vi "Tool Object.vi"(8 "error in (no error)":errorcluster, 11 "Tool Dots in":refnum<class "Tool Dots.lvclass">) -> (0 "error out":errorcluster, 3 "Tool Dots out":refnum<class "Tool Dots.lvclass">)   [LabVIEW 2019, in "Tool Dots.lvclass"]
uses:
  Tool Dots.lvclass
  Settings/ObjectSettings/ObjectSettings.lvclass/ObjectSettings.ctl
  Parse/PathCommands/Point.ctl
  Parse/Dot/Dot.lvclass/Dot.ctl
  Settings/Dot Settings/Dot Settings.lvclass/Dot Settings.ctl
  Parse/Dot/Read cx.vi
  Parse/Dot/Read cy.vi
  Settings/Dot Settings/Dot Settings.lvclass
  C:/Users/Albro/Documents/GitHub/AFM-Lithography/lvsrc/Classes/Settings/ObjectSettings/ObjectSettings.lvclass
  Tool Object/Tool Object.lvclass
  Parse/Dot/Dot.lvclass
  Parse/PathCommands/PathCommands.lvclass
  Settings/ObjectSettings/ObjectSettings.lvclass
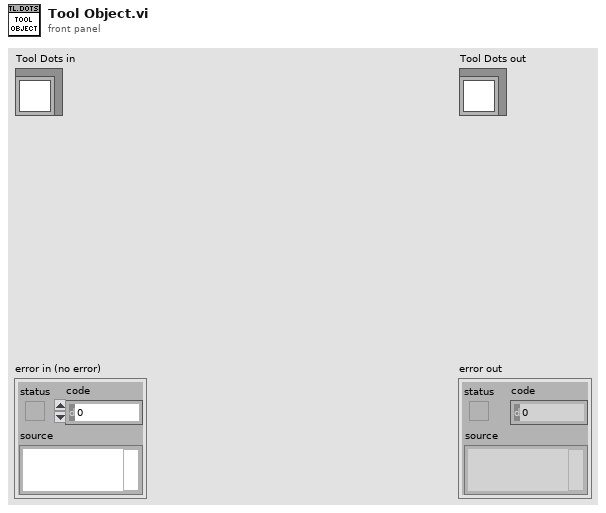
[diagram p1: front panel]
types:
  T1 = typedef "PathCommands.lvclass/Point.ctl" = cluster{"X":dbl, "Y":dbl}
  T2 = typedef "Dot Settings.lvclass/Action.ctl" = enum16{"IV", "QD"}
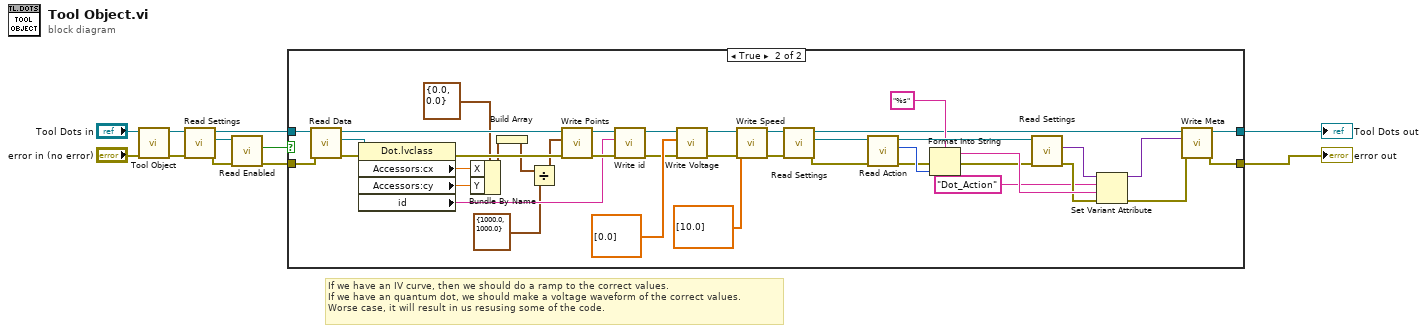
[diagram p0: block diagram]
diagram:
  # "If we have an IV curve, then we should do a ramp to the correct values.\nIf we have an quantum dot, we should make a voltage waveform of the correct values.\nWorse case, it will result in us resusing some of the code."
  n1 = call-parent "Tool Object.vi"("error in (no error)"="error in (no error)", "Tool Object in"="Tool Dots in") -> ("error out"=w7:errorcluster, "Tool Object out"=w9:refnum<class "Tool Dots.lvclass">)  [unwired: 8 in]
  n2 = call-dynamic "Read Settings.vi"("error in (no error)"=w7, "Tool Dots in"=w9) -> ("error out"=w5:errorcluster, "Dot Settings.lvclass"=w6:refnum<class "Dot Settings.lvclass">, "Tool Dots out"=w8:refnum<class "Tool Dots.lvclass">)  [unwired: 7 in]
  n3 = call "Read Enabled.vi"("error in (no error)"=w5, "ObjectSettings in"=w6) -> ("error out"=w4:errorcluster, "Enabled"=w3:bool)  [unwired: 7 in, 1 out]
  n4 = case shown="True" w3 {
    tunnel: w8 -> [w13 w42]
    tunnel: w4 -> [w12 w41]
    tunnel: [w13 w18] -> w2
    tunnel: [w12 w17] -> w1
    frame False {
    }
    frame True {
      n5 = call-dynamic "Read Data.vi"("error in (no error)"=w41, "Tool Dots in"=w42) -> ("error out"=w52:errorcluster, "Dot.lvclass"=w53:refnum<class "Dot.lvclass">, "Tool Dots out"=w51:refnum<class "Tool Dots.lvclass">)  [unwired: 7 in]
      n6 = property class="Dot.lvclass"(reference=w53, error in=w52) -> (error out=w50:errorcluster, "Accessors:cx"=w48:dbl, "Accessors:cy"=w47:dbl, "id"=w43:string)  [unwired: 1 out]
      n7 = Bundle By Name(cluster=T1 {"X"=0.0, "Y"=0.0} ("Point"), "X"=w48, "Y"=w47) -> (w46:T1)
      n8 = Build Array(w46) -> (w15:T1[])
      n9 = Divide(x=w15, y=T1 {"X"=1000.0, "Y"=1000.0} ("Point")) -> (x/y=w14:T1[])
      n10 = call-dynamic "Write Points.vi"("error in (no error)"=w50, "Points"=w14, "Tool Object in"=w51) -> ("error out"=w44:errorcluster, "Tool Object out"=w45:refnum<class "Tool Dots.lvclass">)  [unwired: 7 in]
      n11 = call-dynamic "Write id.vi"("error in (no error)"=w44, "id"=w43, "Tool Object in"=w45) -> ("error out"=w38:errorcluster, "Tool Object out"=w40:refnum<class "Tool Dots.lvclass">)  [unwired: 7 in]
      n12 = call-dynamic "Write Voltage.vi"("error in (no error)"=w38, "Voltage"=dbl[] [0.0], "Tool Object in"=w40) -> ("error out"=w21:errorcluster, "Tool Object out"=w23:refnum<class "Tool Dots.lvclass">)  [unwired: 7 in]
      n13 = call-dynamic "Write Speed.vi"("error in (no error)"=w21, "Speed"=dbl[] [10.0], "Tool Object in"=w23) -> ("error out"=w20:errorcluster, "Tool Object out"=w22:refnum<class "Tool Dots.lvclass">)  [unwired: 7 in]
      n14 = call-dynamic "Read Settings.vi"("error in (no error)"=w20, "Tool Dots in"=w22) -> ("error out"=w24:errorcluster, "Dot Settings.lvclass"=w28:refnum<class "Dot Settings.lvclass">, "Tool Dots out"=w27:refnum<class "Tool Dots.lvclass">)  [unwired: 7 in]
      n15 = call "Read Action.vi"("error in (no error)"=w24, "Dot Settings in"=w28) -> ("error out"=w34:errorcluster, "Action"=w36:T2, "Dot Settings out"=w31:refnum<class "Dot Settings.lvclass">)  [unwired: 7 in]
      n16 = Format Into String(format string="%s", error in=w34, w36) -> (resulting string=w37:string, error out=w35:errorcluster)  [unwired: 1 in]
      n17 = call "Read Settings.vi"("error in (no error)"=w35, "Dot Settings in"=w31) -> ("error out"=w32:errorcluster, "Settings"=w33:variant)  [unwired: 7 in, 1 out]
      n18 = Set Variant Attribute(Variant=w33, name="Dot_Action", value=w37, error in=w32) -> (Variant out=w25:variant, error out=w26:errorcluster)  [unwired: 1 out]
      n19 = call-dynamic "Write Meta.vi"("error in (no error)"=w26, "Meta"=w25, "Tool Object in"=w27) -> ("error out"=w17:errorcluster, "Tool Object out"=w18:refnum<class "Tool Dots.lvclass">)  [unwired: 7 in]
    }
  }
  "error out" <- w1
  "Tool Dots out" <- w2
